vi "Read String.vi"(7 "key":string, 8 "error in (no error)":errorcluster, 9 "default value":string, 11 "TSContext Configuration In":refnum<class "TSContext Configuration.lvclass">) -> (0 "error out":errorcluster, 1 "value":string, 3 "TSContext Configuration Out":refnum<class "TSContext Configuration.lvclass">)   [LabVIEW 2020, in "Astemes_CSVReportPlugin.lvlib" / "TSContext Configuration.lvclass"]
doc: "High-level function for reading configuration file data from process class. If the specified key is not present, it is added with the configured default value."
uses:
  TSContext Configuration.lvclass
  <vilib>/addons/TestStand/_TSUtility.llb/TestStand - Get Property Value (String).vi
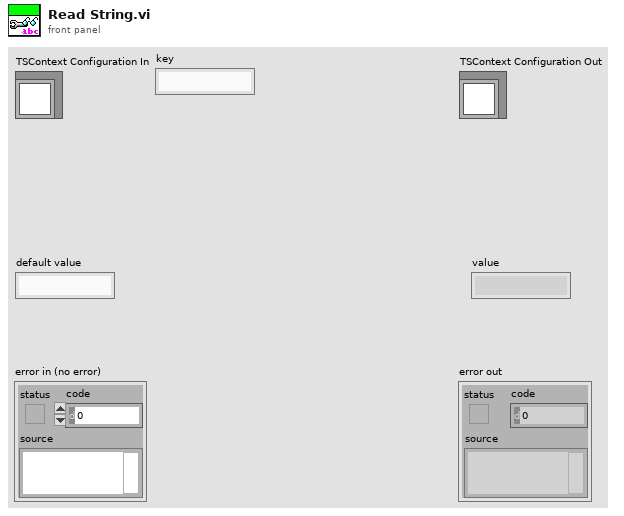
[diagram p1: front panel]
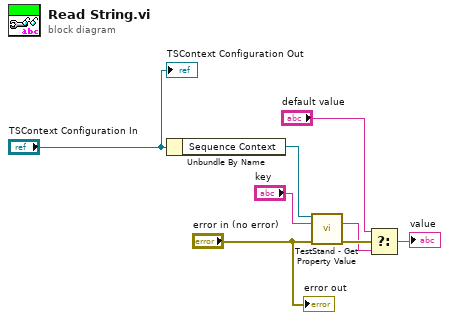
[diagram p0: block diagram]
diagram:
  n1 = Unbundle By Name("TSContext Configuration In") -> ("Sequence Context"=w7:refnum<k7>)
  n2 = call-poly <vilib>:"TestStand - Get Property Value.vi"("Sequence Context In"=w7, "Lookup String"="key", "error in (no error)"="error in (no error)") -> ("Value"=w4:string, "error out"=w8:errorcluster)  [unwired: 10 in, 1 out]
  n3 = Select(t="default value", s=w8, f=w4) -> (s? t:f=→"value":string)
  "error out" <- "error in (no error)"
  "TSContext Configuration Out" <- "TSContext Configuration In"
